vi "formatUpdateJson.vi"(8 "error in (no error)":errorcluster, 10 "Init/Update":bool, 11 "Refnum in":T1) -> (0 "error out":errorcluster, 2 "Update Data":string[](array[string]), 3 "Refnum out":T1)   [LabVIEW 2018]
uses:
  <vilib>/httpClient/ClientHandle.ctl
  <vilib>/Utility/file.llb/Read Delimited Spreadsheet (string).vi
  <vilib>/httpClient/LabVIEWHTTPClient.lvlib
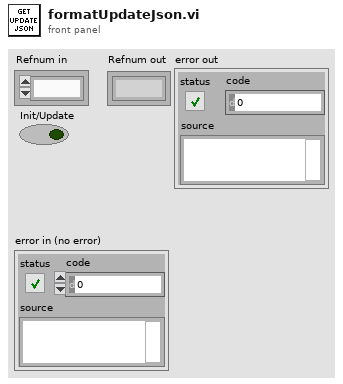
[diagram p1: front panel]
types:
  T1 = typedef "LabVIEWHTTPClient.lvlib/ClientHandle.ctl" = refnum<k1>
  T2 = cluster{"ID":string, "Date":string, "StreetAddress":string, "longitude":string, "latitude":string, "Device":string, "Index":string}[]
  T3 = cluster{"ID":string, "Date":string, "StreetAddress":string, "longitude":string, "latitude":string, "Device":string, "Index":string}
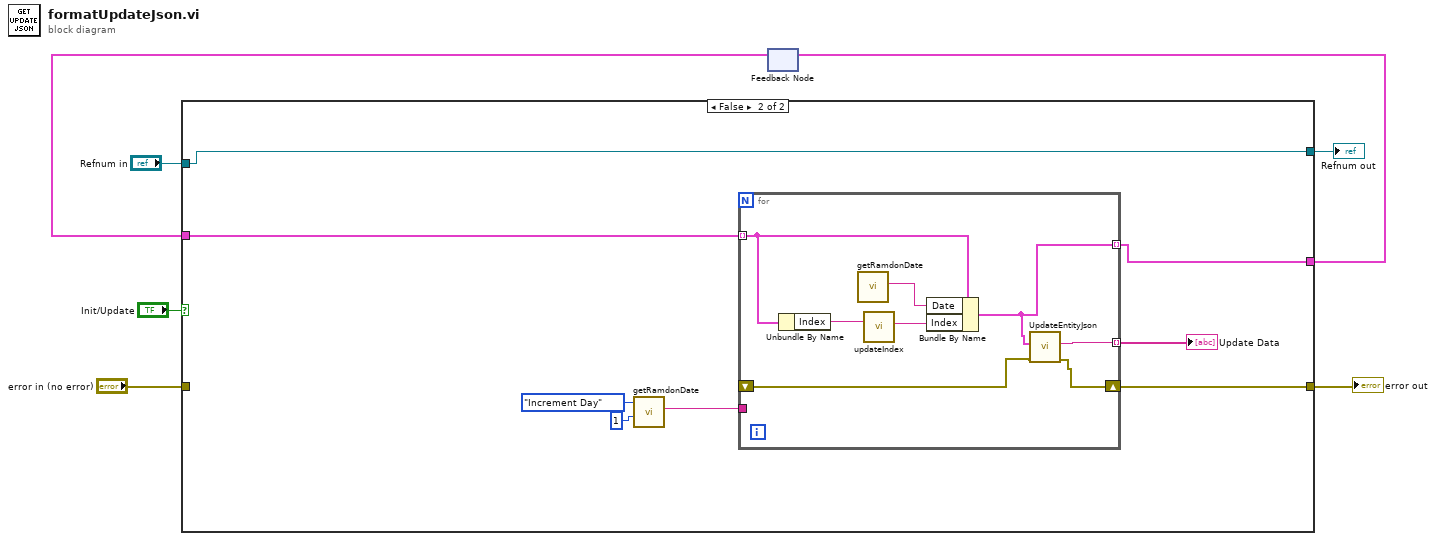
[diagram p0: block diagram]
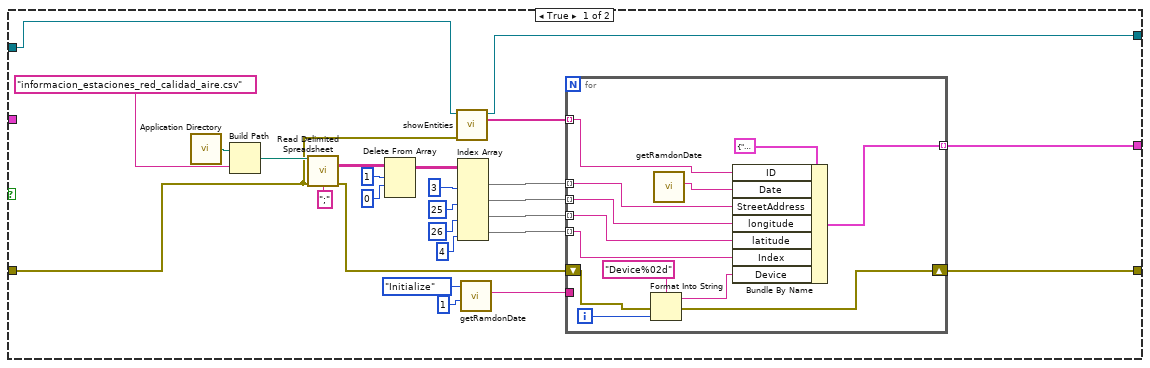
[diagram p2: hidden frame]
diagram:
  n1 = feedback #1() -> (w6:T2)  [unwired: 1 in]
  n2 = case shown="False" "Init/Update" {
    tunnel: [w14 w48] -> w7
    tunnel: w6 -> [_ w51]
    tunnel: [w13 w49] -> w4
    tunnel: "error in (no error)" -> [w11 _]
    tunnel: "Refnum in" -> [w8 w47]
    tunnel: [w9 w47] -> w1
    frame True {
      n3 = call <vilib>:"Application Directory.vi"() -> ("Application Directory"=w24:path)
      n4 = Build Path(base path=w24, name or relative path="informacion_estaciones_red_calidad_aire.csv") -> (appended path=w25:path)
      n5 = call-poly <vilib>:"Read Delimited Spreadsheet.vi"("file path (dialog if empty)"=w25, "error in (no error)"=w11, "delimiter (\\t)"=";" ("delimiter (\\t)")) -> ("all rows"=w30:string[][], "error out"=w15:errorcluster)  [unwired: 7 in, 4 out]
      n6 = Delete From Array(array=w30, length=1, index (row)=0) -> (array with subset deleted=w33:string[][])  [unwired: 1 in, 1 out]
      n7 = call "showEntities.vi"("error in (no error)"=w11, "Refnum in"=w8) -> ("EntitiesList"=w12:string[], "Refnum out"=w9:T1)  [unwired: 7 in, 1 out]
      n8 = Index Array(array=w33, index (col) #1=3 ("disabled index (col)"), index (col) #2=25 ("index (col)"), index (col) #3=26 ("index (col)"), index (col) #4=4 ("index (col)")) -> (element #1=w20:string[], element #2=w19:string[], element #3=w18:string[], element #4=w17:string[])  [unwired: 4 in]
      n9 = call "getRamdonDate.vi"("Start Day"=1, "Action (GetDate)"=enum16{"Initialize", "GetDate", "Increment Day"}."Initialize") -> ("Ramdon date"=w16:string)  [unwired: 9 in]
      n10 = for {
        tunnel: w12 -> [w41] mode=indexing
        tunnel: w20 -> [w40] mode=indexing
        tunnel: w19 -> [w39] mode=indexing
        tunnel: w18 -> [w38] mode=indexing
        tunnel: w17 -> [w37] mode=indexing
        tunnel: w16 -> [_]
        shift-right: [w35] -> w13
        shift-left: w15 -> [w36]
        tunnel: [w34] -> w14 mode=indexing
        i -> [w43]
        n11 = Format Into String(format string="Device%02d", error in=w36, w43) -> (resulting string=w42:string, error out=w35:errorcluster)  [unwired: 1 in]
        n12 = call "getRamdonDate.vi"() -> ("Ramdon date"=w46:string)  [unwired: 11 in]
        n13 = Bundle By Name(cluster=T3 {"ID"="AirQualityUnit24", "Date"="2021-01-1T16:10:27-02:00", "StreetAddress"="Plaza Tres Olivos ", "longitude"="-3.6897308", "latitude"="40.5005477", "Device"="Device24", "Index"="45"} ("Data"), "ID"=w41, "Date"=w46, "StreetAddress"=w40, "longitude"=w39, "latitude"=w38, "Index"=w37, "Device"=w42) -> (w34:T3)
      }
    }
    frame False {
      n14 = call "getRamdonDate.vi"("Start Day"=1, "Action (GetDate)"=enum16{"Initialize", "GetDate", "Increment Day"}."Increment Day") -> ("Ramdon date"=w52:string)  [unwired: 9 in]
      n15 = for {
        tunnel: w51 -> [w61] mode=indexing
        tunnel: w52 -> [_]
        tunnel: [w55] -> w50 mode=indexing
        shift-right: [w56] -> w49
        shift-left: _ -> [w57]
        tunnel: [w58] -> w48 mode=indexing
        n16 = Unbundle By Name(w61) -> ("Index"=w60:string)
        n17 = call "getRamdonDate.vi"() -> ("Ramdon date"=w62:string)  [unwired: 11 in]
        n18 = call "updateIndex.vi"("index"=w60) -> ("new index"=w59:string)  [unwired: 10 in]
        n19 = Bundle By Name(cluster=w61, "Date"=w62, "Index"=w59) -> (w58:T3)
        n20 = call "UpdateEntityJson.vi"("error in (no error)"=w57, "Data"=w58) -> ("error out"=w56:errorcluster, "AirQualityObservedEntity"=w55:string)  [unwired: 8 in]
      }
      "Update Data" <- w50
    }
  }
  "error out" <- w4
  "Refnum out" <- w1
  n21 = feedback-in #1(w7) -> ()
